vi "Eliminated.vi"(6 "Column":i32, 8 "Row":i32, 9 "Killer Index":i32, 10 "Team Index":i32, 11 "Atomic in":refnum<class "Atomic.lvclass">) -> (3 "Atomic out":refnum<class "Atomic.lvclass">)   [LabVIEW 2017, in "Atomic.lvclass"]
uses:
  Atomic.lvclass
  Square/Square.lvclass
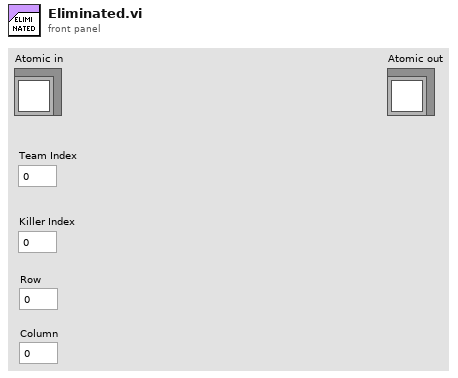
[diagram p1: front panel]
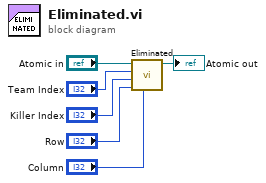
[diagram p0: block diagram]
diagram:
  n1 = call-parent "Eliminated.vi"("Column"="Column", "Row"="Row", "Killer Index"="Killer Index", "Team Index"="Team Index", "Square in"="Atomic in") -> ("Square out"=→"Atomic out":refnum<class "Atomic.lvclass">)  [unwired: 6 in]
